vi "Array 2.vi"() -> ()   [LabVIEW 2011]
panel:
  out "Output":dbl[](array[numeric])
  in  "index":dbl
  in  "Sub Array":dbl[](array[numeric])
  in  "Input":dbl[](array[numeric])
  out "Min Index":dbl
  out "Max Index":dbl
  out "Min Value":dbl
  out "Max Value":dbl
  in  "Array 2":dbl[](array[numeric])
  in  "index":dbl
  in  "element":dbl
  out "output":dbl
  in  "Array":dbl[](array[numeric])
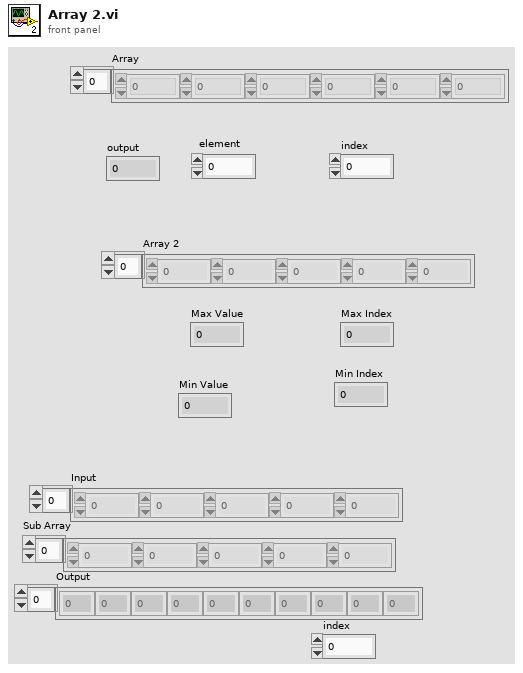
[diagram p1: front panel]
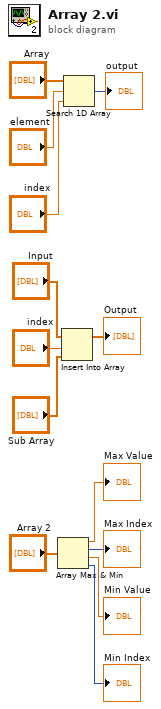
[diagram p0: block diagram]
diagram:
  n1 = Array Max & Min(array="Array 2") -> (max value=→"Max Value":dbl, max index (indices)=→"Max Index":i32, min value=→"Min Value":dbl, min index (indices)=→"Min Index":i32)
  n2 = Insert Into Array(array="Input", index="index", new element="Sub Array") -> (→"Output":dbl[])
  n3 = Search 1D Array(1D array="Array", element="element", start index (0)="index") -> (index of element=→"output":i32)
